vi "Settings_init.vi"() -> ()   [LabVIEW 2009]
panel:
  out "appended path":path
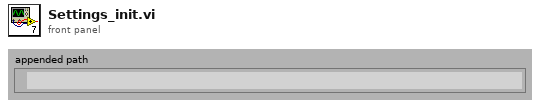
[diagram p1: front panel]
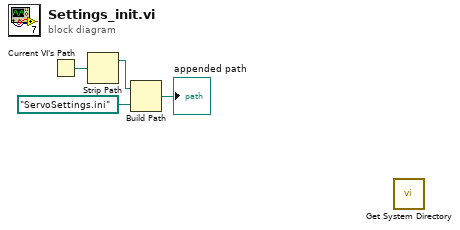
[diagram p0: block diagram]
diagram:
  n1 = Current VI's Path() -> (path=w2:path)
  n2 = Strip Path(path=w2) -> (stripped path=w1:path)  [unwired: 1 out]
  n3 = Build Path(base path=w1, name or relative path=path "ServoSettings.ini" ("configuration file path")) -> (appended path=→"appended path":path)
  n4 = call <vilib>:"Get System Directory.vi"() -> ()  [unwired: 11 in, 1 out]
